vi "SplitDMAFIFOData.vi"(8 "error in (no error)":errorcluster, 11 "Data Array IN":u64[](array[numeric])) -> (0 "error out":errorcluster, 1 "Image trig":u16[](array[numeric]), 2 "Time at P_final if less than t_final":u32[](array[numeric]), 3 "Final step, n":u16[](array[numeric]))   [LabVIEW 2016]
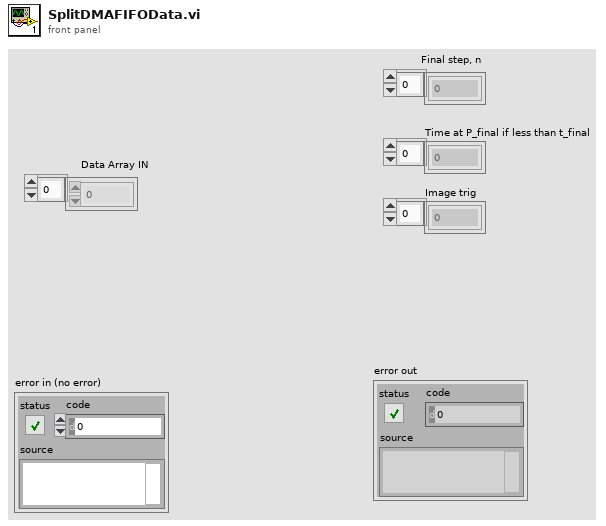
[diagram p1: front panel]
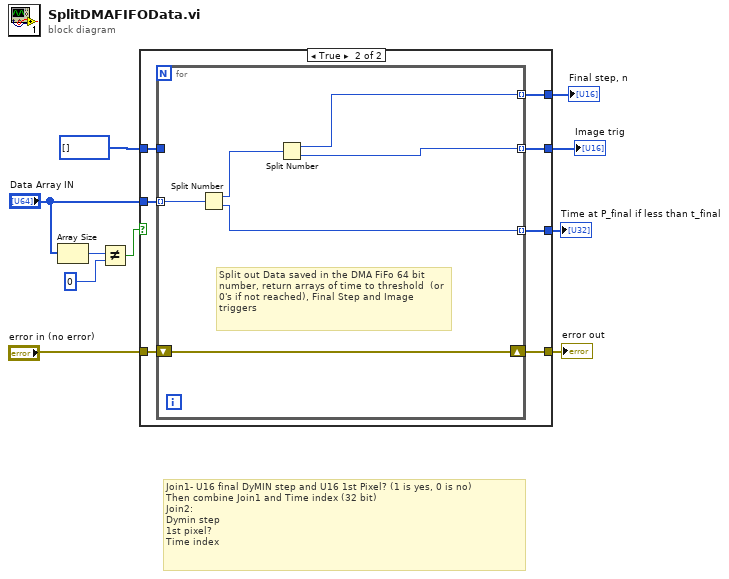
[diagram p0: block diagram]
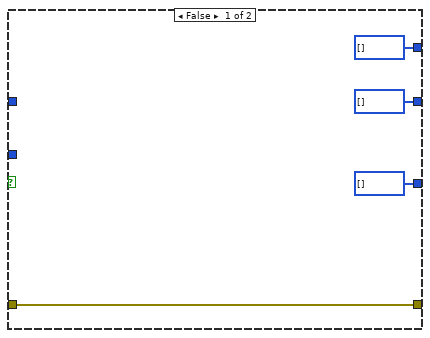
[diagram p2: hidden frame]
diagram:
  # "Join1- U16 final DyMIN step and U16 1st Pixel? (1 is yes, 0 is no)\nThen combine Join1 and Time index (32 bit)\nJoin2:\nDymin step\n1st pixel?\nTime index"
  n1 = Array Size(array="Data Array IN") -> (size(s)=w7:i32)
  n2 = Not Equal?(x=w7, y=0) -> (x != y?=w5:bool)
  n3 = case shown="True" w5 {
    tunnel: "error in (no error)" -> [w11 w21]
    tunnel: u16[] [] -> [_ w20]
    tunnel: "Data Array IN" -> [_ w19]
    tunnel: [u16[] [] w18] -> w4
    tunnel: [u16[] [] w17] -> w3
    tunnel: [u32[] [] w16] -> w2
    tunnel: [w11 w15] -> w1
    frame False {
    }
    frame True {
      n4 = for {
        tunnel: w19 -> [w26] mode=indexing
        shift-right: [w27] -> w15
        shift-left: w21 -> [w27]
        tunnel: [w25] -> w16 mode=indexing
        tunnel: [w23] -> w18 mode=indexing
        tunnel: w20 -> [_]
        tunnel: [w22] -> w17 mode=indexing
        # "Split out Data saved in the DMA FiFo 64 bit number, return arrays of time to threshold  (or 0's if not reached), Final Step and Image triggers"
        n5 = Split Number(x=w26) -> (hi(x)=w24:u32, lo(x)=w25:u32)
        n6 = Split Number(x=w24) -> (hi(x)=w23:u16, lo(x)=w22:u16)
      }
    }
  }
  "Final step, n" <- w4
  "Image trig" <- w3
  "Time at P_final if less than t_final" <- w2
  "error out" <- w1
